vi "ID_Regulering.vi"(8 "k_d":dbl, 9 "k_i":dbl, 10 "SP":dbl, 11 "DATA":dbl) -> (0 "d_id":dbl, 1 "i_id":dbl, 2 "e(t)":dbl, 3 "u_id":dbl)   [LabVIEW 2022 SP3]
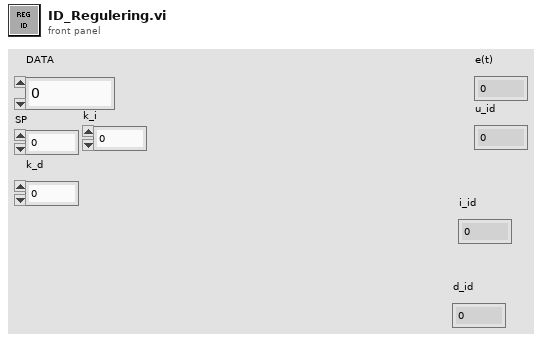
[diagram p1: front panel]
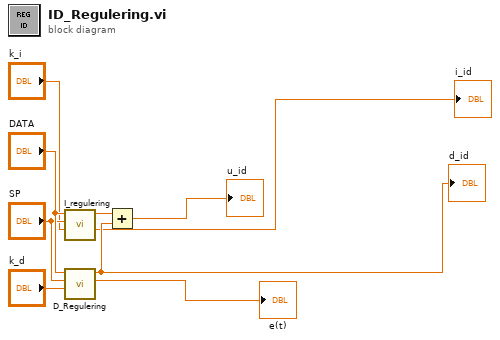
[diagram p0: block diagram]
diagram:
  n1 = call "I_regulering.vi"("k_i"="k_i", "SP"="SP", "DATA"="DATA") -> ("i_i"=→"i_id":dbl, "u_i"=w4:dbl)  [unwired: 6 in, 1 out]
  n2 = call "D_Regulering.vi"("k_d"="k_d", "SP"="SP", "DATA"="DATA") -> ("e(t)"=→"e(t)":dbl, "u_d"=w2:dbl)  [unwired: 7 in]
  "d_id" <- w2
  n3 = Add(x=w4, y=w2) -> (x+y=→"u_id":dbl)
